vi "PreviewMessage.vi"(7 "Timeout (-1 ms)":i32=-1, 8 "error in (no error)":errorcluster, 11 "MessageQueue":refnum<class "MessageQueue.lvclass">) -> (0 "error out":errorcluster, 1 "Message out":refnum<class "Message.lvclass">, 2 "Message Name":string, 3 "MessageQueue out":refnum<class "MessageQueue.lvclass">, 4 "Timed Out?":bool)   [LabVIEW 2009, in "LapDog.Messaging.v2.lvlib" / "MessageQueue.lvclass"]
doc: "Returns a copy the first message in the message queue. The original message remains in the queue.\n\nThis method returns one of three standard messages under the following conditions:\n-A \"QueueTimeoutMessage\" Message object is returned if the timeout expires.\n-A \"QueueErrorInMessage\" ErrorMessage object is returned if an error is present on the error in terminal.\n-A \"QueueErrorMessage\" ErrorMessage object is returned if an error occurs during the preview operation.\n\nThis method clears all errors and warnings from the error wire before returning."
uses:
  MessageQueue.lvclass
  MessageObject/Message.lvclass
  MessageQueue.lvclass/MessageQueue.ctl
  ErrorMessage/ErrorMessage.lvclass
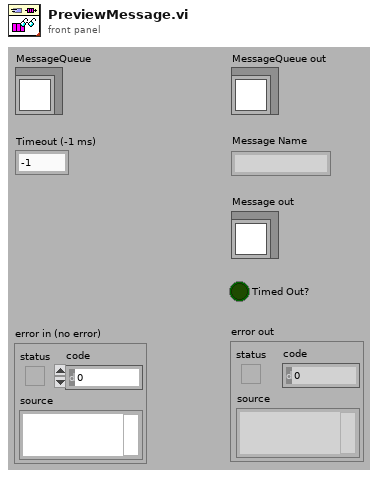
[diagram p1: front panel]
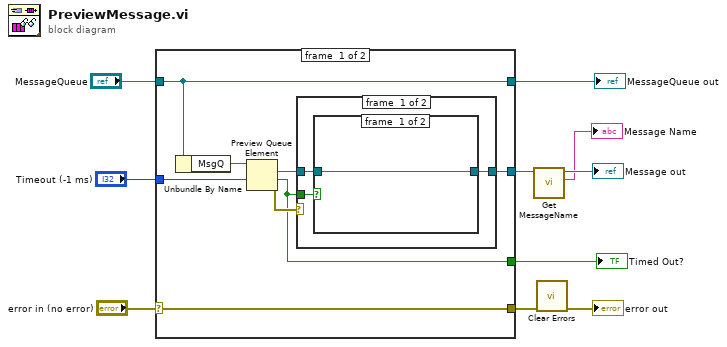
[diagram p0: block diagram]
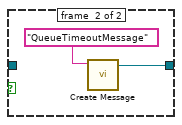
[diagram p2: hidden frame]
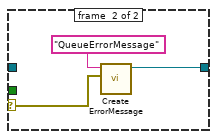
[diagram p3: hidden frame]
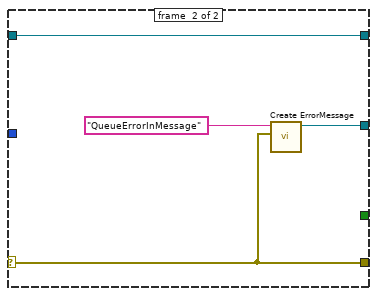
[diagram p4: hidden frame]
diagram:
  n1 = case shown="Error" "error in (no error)" {
    selector: "error in (no error)" -> [w12 w29]
    tunnel: [w17 w30] -> w3
    tunnel: "Timeout (-1 ms)" -> [w16 _]
    tunnel: "MessageQueue" -> [w14 w31]
    tunnel: [w12 w29] -> w4
    tunnel: [w14 w31] -> w2
    tunnel: [w11 _] -> w1
    frame #0 {
      n2 = Unbundle By Name(w14) -> ("MsgQ"=w15:refnum<queue>)
      n3 = Preview Queue Element(queue=w15, timeout in ms (-1)=w16) -> (element=w18:refnum<class "Message.lvclass">, timed out?=w11:bool, error out=w13:errorcluster)  [unwired: 1 in, 1 out]
      n4 = case shown="No Error" w13 {
        selector: w13 -> [_ w26]
        tunnel: w18 -> [w19 _]
        tunnel: [w20 w27] -> w17
        tunnel: w11 -> [w21 _]
        frame #0 {
          n5 = case shown="True" w21 {
            tunnel: [w22 w23] -> w20
            tunnel: w19 -> [w22 _]
            frame #0 {
            }
            frame #1 {
              n6 = call "Create Message.vi"("Message Name"="QueueTimeoutMessage") -> ("Message out"=w23:refnum<class "Message.lvclass">)  [unwired: 9 in, 1 out]
            }
          }
        }
        frame #1 {
          n7 = call "Create ErrorMessage.vi"("Error Cluster"=w26, "Message Name"="QueueErrorMessage") -> ("ErrorMessage out"=w27:refnum<class "ErrorMessage.lvclass">)  [unwired: 8 in, 1 out]
        }
      }
    }
    frame #1 {
      n8 = call "Create ErrorMessage.vi"("Error Cluster"=w29, "Message Name"="QueueErrorInMessage") -> ("ErrorMessage out"=w30:refnum<class "ErrorMessage.lvclass">)  [unwired: 8 in, 1 out]
    }
  }
  "MessageQueue out" <- w2
  "Timed Out?" <- w1
  n9 = call "Get MessageName.vi"("Message in"=w3) -> ("Message Name"=→"Message Name":string, "Message out"=→"Message out":refnum<class "Message.lvclass">)  [unwired: 1 in, 8 out]
  n10 = call <vilib>:"Clear Errors.vi"("error in (no error)"=w4) -> ("error out"=→"error out":errorcluster)  [unwired: 6 out]
